vi "verify acquisition status.vi"(8 "error in (no error)":errorcluster, 11 "Channel in":refnum<class "Channel.lvclass">) -> (0 "error out":errorcluster, 2 "acq status":cluster{"frames":bool, "cycles":bool}, 3 "Channel out":refnum<class "Channel.lvclass">)   [LabVIEW 2018, in "Channel.lvclass"]
uses:
  Channel.lvclass
  Channel.lvclass/Channel.ctl
  Camera/Camera.lvclass
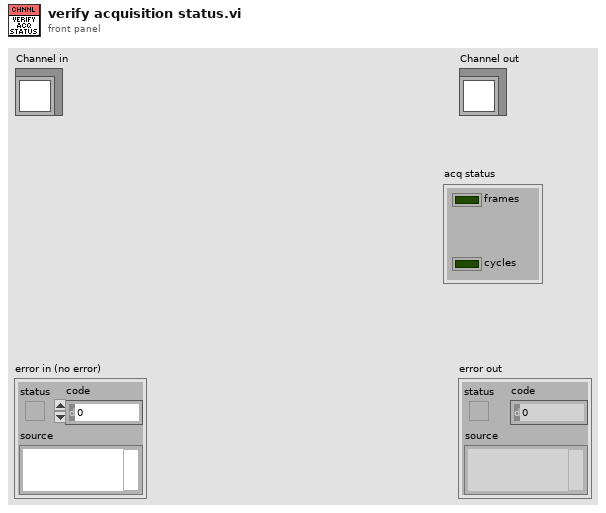
[diagram p1: front panel]
types:
  T1 = cluster{"CYCLES_DONE":u16, "LAST_IMAGE_NAME":string, "USED_DISK_SPACE":u16, "FRAMES_DONE":u16, "CCD_STATUS":string, "CURRENT_TEMPERATURE":i16, "TEMPERATURE_STATUS":string, "FRAME_EXPOSURE_TIME":sgl, "ERROR":bool, "SERIAL_NUMBER":u16, "ACQUIRING":bool, "IMAGE_INDEX":u32, "power":bool, "acs mode":bool}
  T2 = cluster{"EXPTIME":dbl, "#FRAMES":u32, "#CYCLES":u32, "suffix":string, "TEMP":i32, "COOLER_POWER_STATUS":u16}
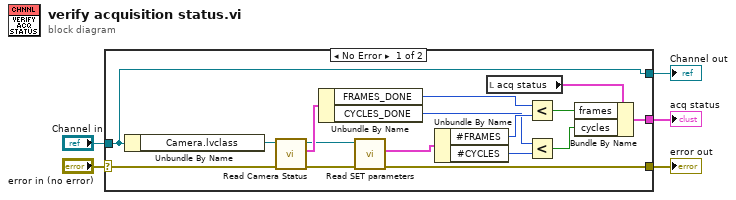
[diagram p0: block diagram]
diagram:
  n1 = case shown="No Error" "error in (no error)" {
    selector: "error in (no error)" -> [w13 w23]
    tunnel: [w15 w23] -> w4
    tunnel: [w21 w22] -> w2
    tunnel: "Channel in" -> [w21 w22]
    tunnel: [w8 _] -> w1
    frame No Error {
      n2 = Unbundle By Name(w21) -> ("Camera.lvclass"=w12:refnum<class "Camera.lvclass">)
      n3 = call-dynamic "Read Camera Status.vi"("error in (no error)"=w13, "Camera in"=w12) -> ("error out"=w16:errorcluster, "Camera Status"=w19:T1, "Camera out"=w14:refnum<class "Camera.lvclass">)  [unwired: 7 in]
      n4 = Unbundle By Name(w19) -> ("FRAMES_DONE"=w18:u16, "CYCLES_DONE"=w11:u16)
      n5 = call-dynamic "Read SET parameters.vi"("error in (no error)"=w16, "Camera in"=w14) -> ("error out"=w15:errorcluster, "SET parameters"=w20:T2)  [unwired: 7 in, 1 out]
      n6 = Unbundle By Name(w20) -> ("#FRAMES"=w17:u32, "#CYCLES"=w10:u32)
      n7 = local read "acq status"() -> (w9:cluster{"frames":bool, "cycles":bool})
      n8 = Less?(x=w18, y=w17) -> (x < y?=w7:bool)
      n9 = Less?(x=w11, y=w10) -> (x < y?=w6:bool)
      n10 = Bundle By Name(cluster=w9, "frames"=w7, "cycles"=w6) -> (w8:cluster{"frames":bool, "cycles":bool})
    }
    frame Error {
    }
  }
  "error out" <- w4
  "Channel out" <- w2
  "acq status" <- w1
